vi "Commands.vi"(0 "Final Output":T1, 1 "Other Outputs":cluster{"Alarm":bool, "Heater":bool}) -> (2 "Commands":bool[](array[boolean]), 3 "hex integer string":string, 4 "number":u32)   [LabVIEW 2013]
uses:
  Type Defs/Final Output.ctl
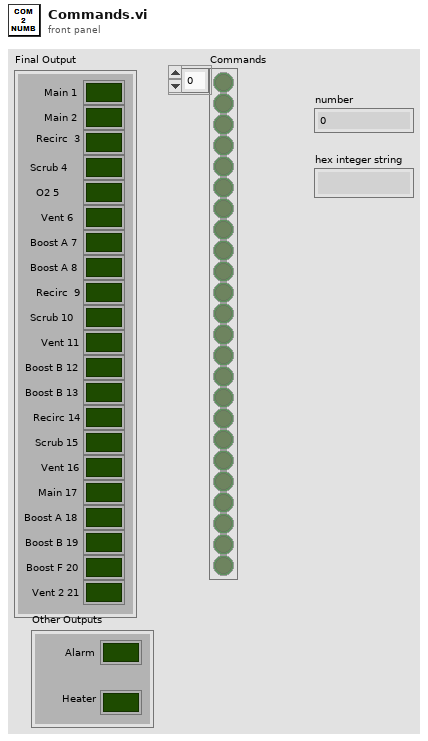
[diagram p1: front panel]
types:
  T1 = typedef "Final Output.ctl" = cluster{"Main 1":bool, "Main 2":bool, "Recirc  3":bool, "Scrub 4":bool, "O2 5":bool, "Vent 6":bool, "Boost A 7":bool, "Boost A 8":bool, "Recirc  9":bool, "Scrub 10":bool, "Vent 11":bool, "Boost B 12":bool, "Boost B 13":bool, "Recirc 14":bool, "Scrub 15":bool, "Vent 16":bool, "Main 17":bool, "Boost A 18":bool, "Boost B 19":bool, "Boost F 20":bool, "Vent 2 21":bool}
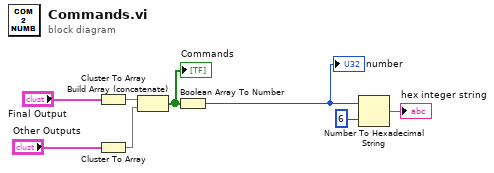
[diagram p0: block diagram]
diagram:
  n1 = Cluster To Array(cluster="Final Output") -> (array=w6:bool[])
  n2 = Cluster To Array(cluster="Other Outputs") -> (array=w5:bool[])
  n3 = Build Array (concatenate)(w6, w5) -> (w4:bool[])
  "Commands" <- w4
  n4 = Boolean Array To Number(Boolean array=w4) -> (number=w2:u32)
  "number" <- w2
  n5 = Number To Hexadecimal String(1:6 ("number"), 2:w2) -> (0:→"hex integer string":string)
